vi "CSMP-Async Call.vi"(0 "State":string, 1 "Args":string, 2 "Source/target":string, 5 "Error In":errorcluster caption="error in (no error)", 8 "Module Name":string, 10 "Msg Type":T1) -> (14 "State Out":string, 15 "Args Out":string, 16 "Source/target Out":string, 17 "Pre-State Out":string, 18 "Pre-Args Out":string, 19 "Error":errorcluster)   [LabVIEW 2017, in "Communicable State Machine.lvlib"]
doc: "### CSMP-Async Call.vi\n\n-- <b>Controls</b> --\n- <b>state</b>:\n- <b>args</b>:\n- <b>source/target</b>:\n- <b>Module Name</b>:\n- <b>Msg Type</b>:\n\n-- <b>Indicators</b> --\n- <b>state out</b>:\n- <b>args out</b>:\n- <b>source/target out</b>:\n- <b>Pre-State out</b>:\n- <b>Pre-Args out</b>:\n- <b>error</b>:"
uses:
  Communicable State Machine.lvlib
  Typedef/_CSM_MSG_TYPE.ctl
  Typedef/_Cross CSM State Data.ctl
  Typedef/_Cross CSM State Response.ctl
  Typedef/_CSM_Response Source Message.ctl
  _Shared/CSM - System States.vi
  Priority Queue/Enqueue Element.vi
  Error/CSM Not Allowed Message.vi
  CSMQ/_CSMOFGV(lvlibp).vi
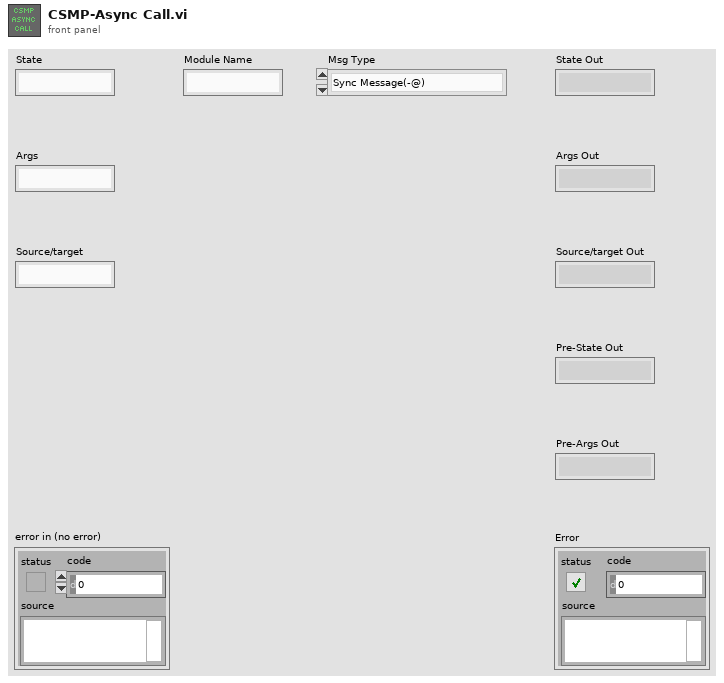
[diagram p1: front panel]
types:
  T1 = typedef "Communicable State Machine.lvlib/_CSM_MSG_TYPE.ctl" = enum16{"Sync Message(-@)", "Async Message(->)", "Async without Response(->|)", "Async Response", "Broadcast(-><all>)", "Broadcast(-><status>)", "Broadcast(-><interrupt>)", "Append to JKISM States", "Append to JKISM States(High Priority)", "Broadcast(-><state>)"}
  T2 = typedef "Communicable State Machine.lvlib/_CSMObj.ctl" = cluster{"info":T3, "Refs":T5}
  T3 = typedef "Communicable State Machine.lvlib/_CSMObj-Info.ctl" = cluster{"Module Name":string, "Requested Name":string, "Group Name":string, "Mode":T4, "Allowed Messages":string[]}
  T4 = typedef "Communicable State Machine.lvlib/_CSM_MODE.ctl" = enum16{"Not Exist", "Stand Alone", "CSM", "Worker", "Worker Agent", "Chain Node", "Chain"}
  T5 = typedef "Communicable State Machine.lvlib/_CSMObj-Refs.ctl" = cluster{"WatchDogQ":refnum<queue>, "CSMDataDVR":refnum<data-value>, "Queue":T6, "GroupDataDVR":refnum<data-value>, "TagMap":refnum<data-value>, "ExitEvent":refnum<user-event>, "NewStateEvent":refnum<user-event>, "StatusChangeEvent":refnum<user-event>}
  T6 = typedef "Communicable State Machine.lvlib/Priority Queue.ctl" = cluster{"HPriorityQ":refnum<queue>, "LowPriorityQ":refnum<queue>}
  T7 = typedef "Communicable State Machine.lvlib/_Cross CSM State Data.ctl" = cluster{"Msg Type":T1, "state":string, "args":string, "source":string, "RespQ":refnum<queue>, "Response For Message":T8, "Target":string}
  T8 = typedef "Communicable State Machine.lvlib/_CSM_Response Source Message.ctl" = cluster{"‘State":string, "’Arguments":string, "’Error":errorcluster}
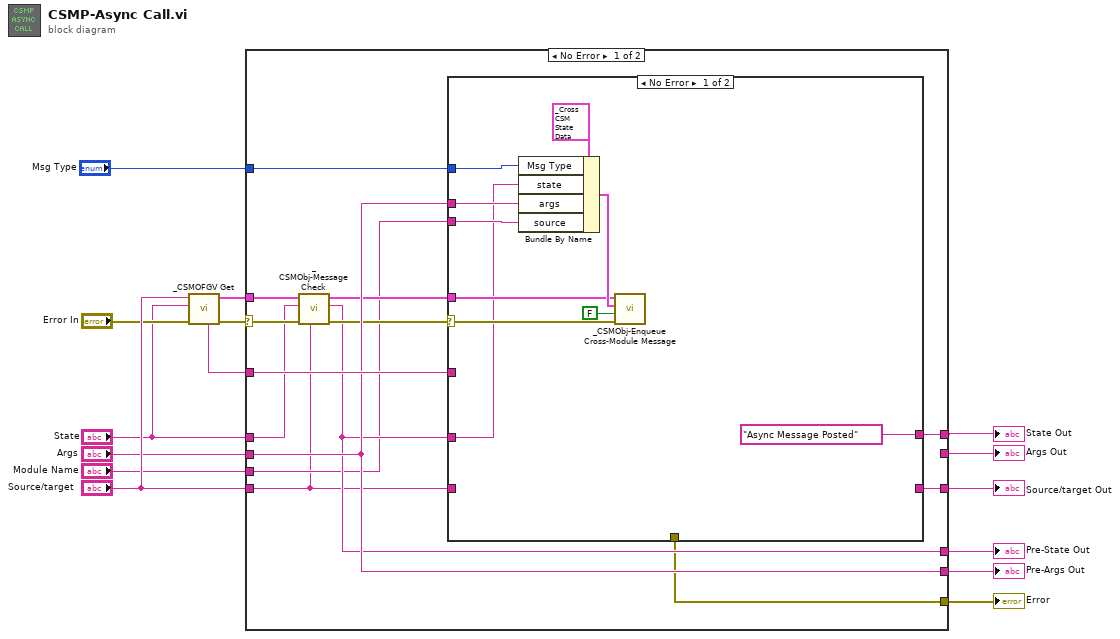
[diagram p0: block diagram]
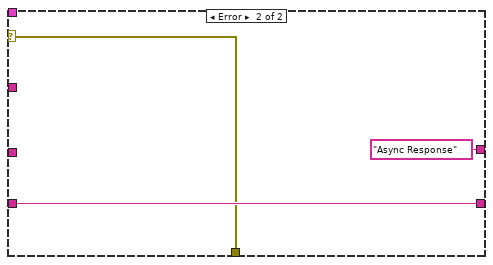
[diagram p2: hidden frame]
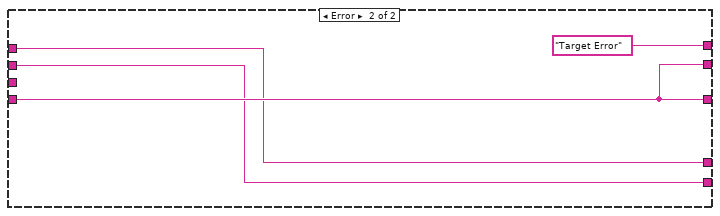
[diagram p3: hidden frame]
diagram:
  n1 = call "_CSMOFGV Get.vi"("Error In"="Error In", "Message"="State", "Name (\"\" to Use UUID) In"="Source/target") -> ("error out"=w15:errorcluster, "CSM-Obj"=w13:T2, "Name"=w14:string)  [unwired: 6 in]
  n2 = case shown="No Error" w15 {
    selector: w15 -> [w23 _]
    tunnel: w13 -> [w24 _]
    tunnel: [w29 "Target Error" ("before match")] -> w9
    tunnel: [_ w45] -> w8
    tunnel: "Source/target" -> [w16 w45]
    tunnel: "State" -> [w20 w44]
    tunnel: "Args" -> [w26 w43]
    tunnel: "Module Name" -> [w17 _]
    tunnel: w14 -> [w28 _]
    tunnel: [w27 w45] -> w7
    tunnel: [w19 w44] -> w5
    tunnel: [w26 w43] -> w4
    tunnel: "Msg Type" -> [w25 _]
    tunnel: [w18 _] -> w2
    frame No Error {
      n3 = call "_CSMObj-Message Check.vi"("CSM"=w16, "Error In"=w23, "Message"=w20, "CSMQ In"=w24) -> ("error out"=w22:errorcluster, "Message (Dup)"=w19:string, "CSMQ Out"=w21:T2)  [unwired: 5 in]
      n4 = case shown="No Error" w22 {
        selector: w22 -> [w32 w40]
        tunnel: w17 -> [w38 _]
        tunnel: ["Async Message Posted" ("before match") "Async Response" ("f")] -> w29
        tunnel: w28 -> [_ _]
        tunnel: w16 -> [_ w42]
        tunnel: [_ w42] -> w27
        tunnel: w26 -> [w34 _]
        tunnel: w25 -> [w33 _]
        tunnel: w21 -> [w31 _]
        tunnel: w19 -> [w30 _]
        tunnel: [_ w40] -> w18
        frame No Error {
          n5 = Bundle By Name(cluster=T7 {"Msg Type"=enum."Sync Message(-@)", "state"="", "args"="", "source"="", "RespQ"=refnum, "Response For Message"={"‘State"="", "’Arguments"="", "’Error"={"status"=FALSE, "code"=0, "source"=""}}, "Target"=""} ("Cross JKI State Machine State"), "Msg Type"=w33, "state"=w30, "args"=w34, "source"=w38) -> (w37:T7)
          n6 = call "_CSMObj-Enqueue Cross-Module Message.vi"("Error In"=w32, "High Priority? (F)"=FALSE ("High Priority?(F)"), "Data"=w37, "CSMQ In"=w31) -> ()  [unwired: 6 in, 2 out]
        }
        frame Error {
        }
      }
    }
    frame Error {
    }
  }
  "State Out" <- w9
  "Args Out" <- w8
  "Source/target Out" <- w7
  "Pre-State Out" <- w5
  "Pre-Args Out" <- w4
  "Error" <- w2
